vi "PXI_Host_U16_Read_NewMethod_Benchmark.vi"() -> ()   [LabVIEW 2018]
uses:
  <vilib>/Platform/TimedLoop/XDataNode/timing_clust.ctl
  <vilib>/Platform/TimedLoop/XDataNode/nitl_modes.ctl
  <vilib>/Platform/TimedLoop/XDataNode/wakeup.ctl
  cRIO RT/FPGA Bitfile Register Operations/Scalar IO Operations/Read Methods/Read Data Register/Instances/Read U16.vi
  cRIO RT/FPGA Bitfile Register Operations/Scalar IO Operations/Utilities/Find Register Offset.vi
  cRIO RT/FPGA Bitfile Register Operations/Scalar IO Operations/SubVIs/Check Register Data Store.vi
  cRIO RT/FPGA Bitfile Register Operations/Scalar IO Operations/Error Handling/Error 6001.vi
  cRIO RT/FPGA Bitfile Register Operations/Scalar IO Operations/Error Handling/Error 6000.vi
  cRIO RT/FPGA Bitfile Register Operations/Scalar IO Operations/Error Handling/Error 6002.vi
  cRIO RT/FPGA Bitfile Register Operations/Scalar IO Operations/Error Handling/Error 6003.vi
  <vilib>/FPGAPlugInAG/Dynamic/niLvFpga_Close_Dynamic.vi
  <vilib>/platform/TimedLoop/XDataNode/XDataNode.xnode
  <vilib>/rvi/interface/nirviCloseFPGA/nirviCloseFPGA.xnode
  cRIO RT/FPGA Bitfile Register Operations/Scalar IO Operations/FPGA Register IO.lvlib
  <vilib>/Platform/TimedLoop/XDataNode/XDNodeRunTimeDep.lvlib
panel:
  out "Standard Dev":dbl
  out "Execution time (s)":dbl
  out "Maximum(s)":dbl
  out "Waveform Graph":dbl[](graph)
  out "Value out":i8
  out "error out":errorcluster
  # "Recorded time"
  # "3.37551E-5"
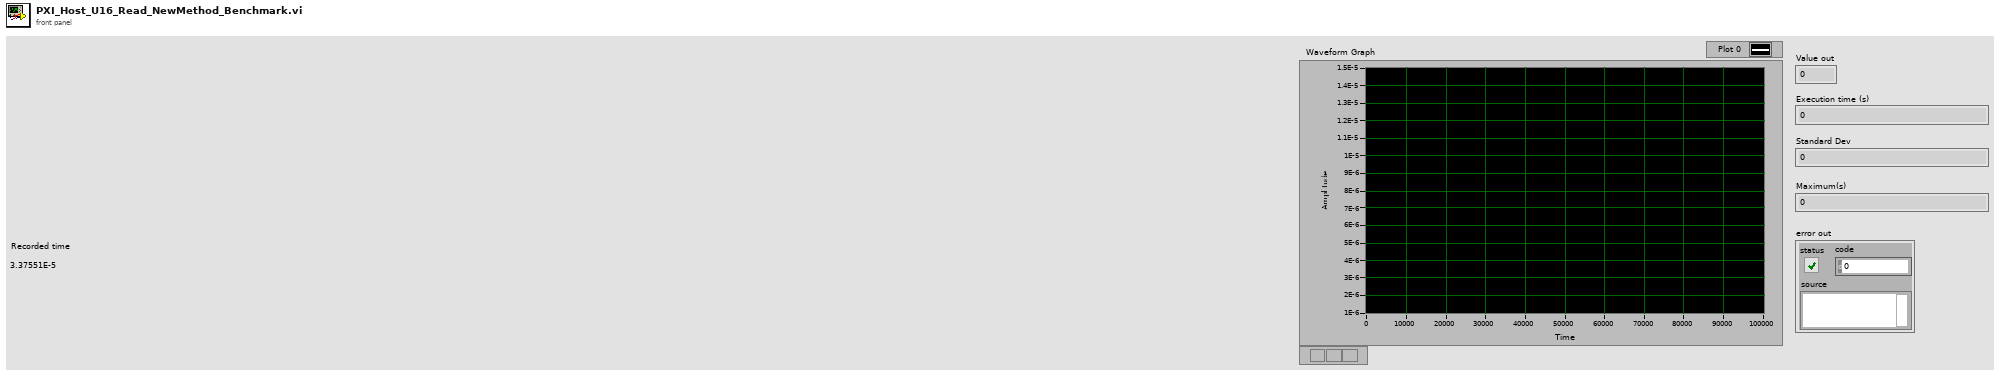
[diagram p1: front panel]
types:
  T1 = typedef "XDNodeRunTimeDep.lvlib/timing_clust.ctl" = cluster{"Expected End [f-1]":u64, "Actual End [f-1]":u64, "Finished Late? [f-1]":bool, "Expected End [i-1]":u64, "Actual End [i-1]":u64, "Finished Late? [i-1]":bool, "Expected Start [i]":u64, "Actual Start [i]":u64, "Expected Start [f]":u64, "Actual Start [f]":u64, "Source Name":string, "Structure Name":string, "Period":i64, "Deadline":i64, "Offset":i64, "Start":i64, "Priority":i32, "Timeout":i32, "Mode":T2, "Wakeup Reason":T3, "Error":errorcluster, "Source Type":string, "Secondary Source Type":string, "Global End Time":u64, "Global Start Time":u64, "Frame Duration":u64, "Iteration Duration":u64, "Assigned CPU":i32, "I/O Scan Engine Mode":u32}
  T2 = typedef "XDNodeRunTimeDep.lvlib/nitl_modes.ctl" = enum32{"No Change", "Process missed periods, maintain original phase", "Discard missed periods, maintain original phase", "Process missed periods, ignore original phase", "Discard missed periods, ignore original phase"}
  T3 = typedef "XDNodeRunTimeDep.lvlib/wakeup.ctl" = enum32{"Normal", "Aborted", "Asynchronous wakeup", "Timing source error", "Timed loop error", "Timeout"}
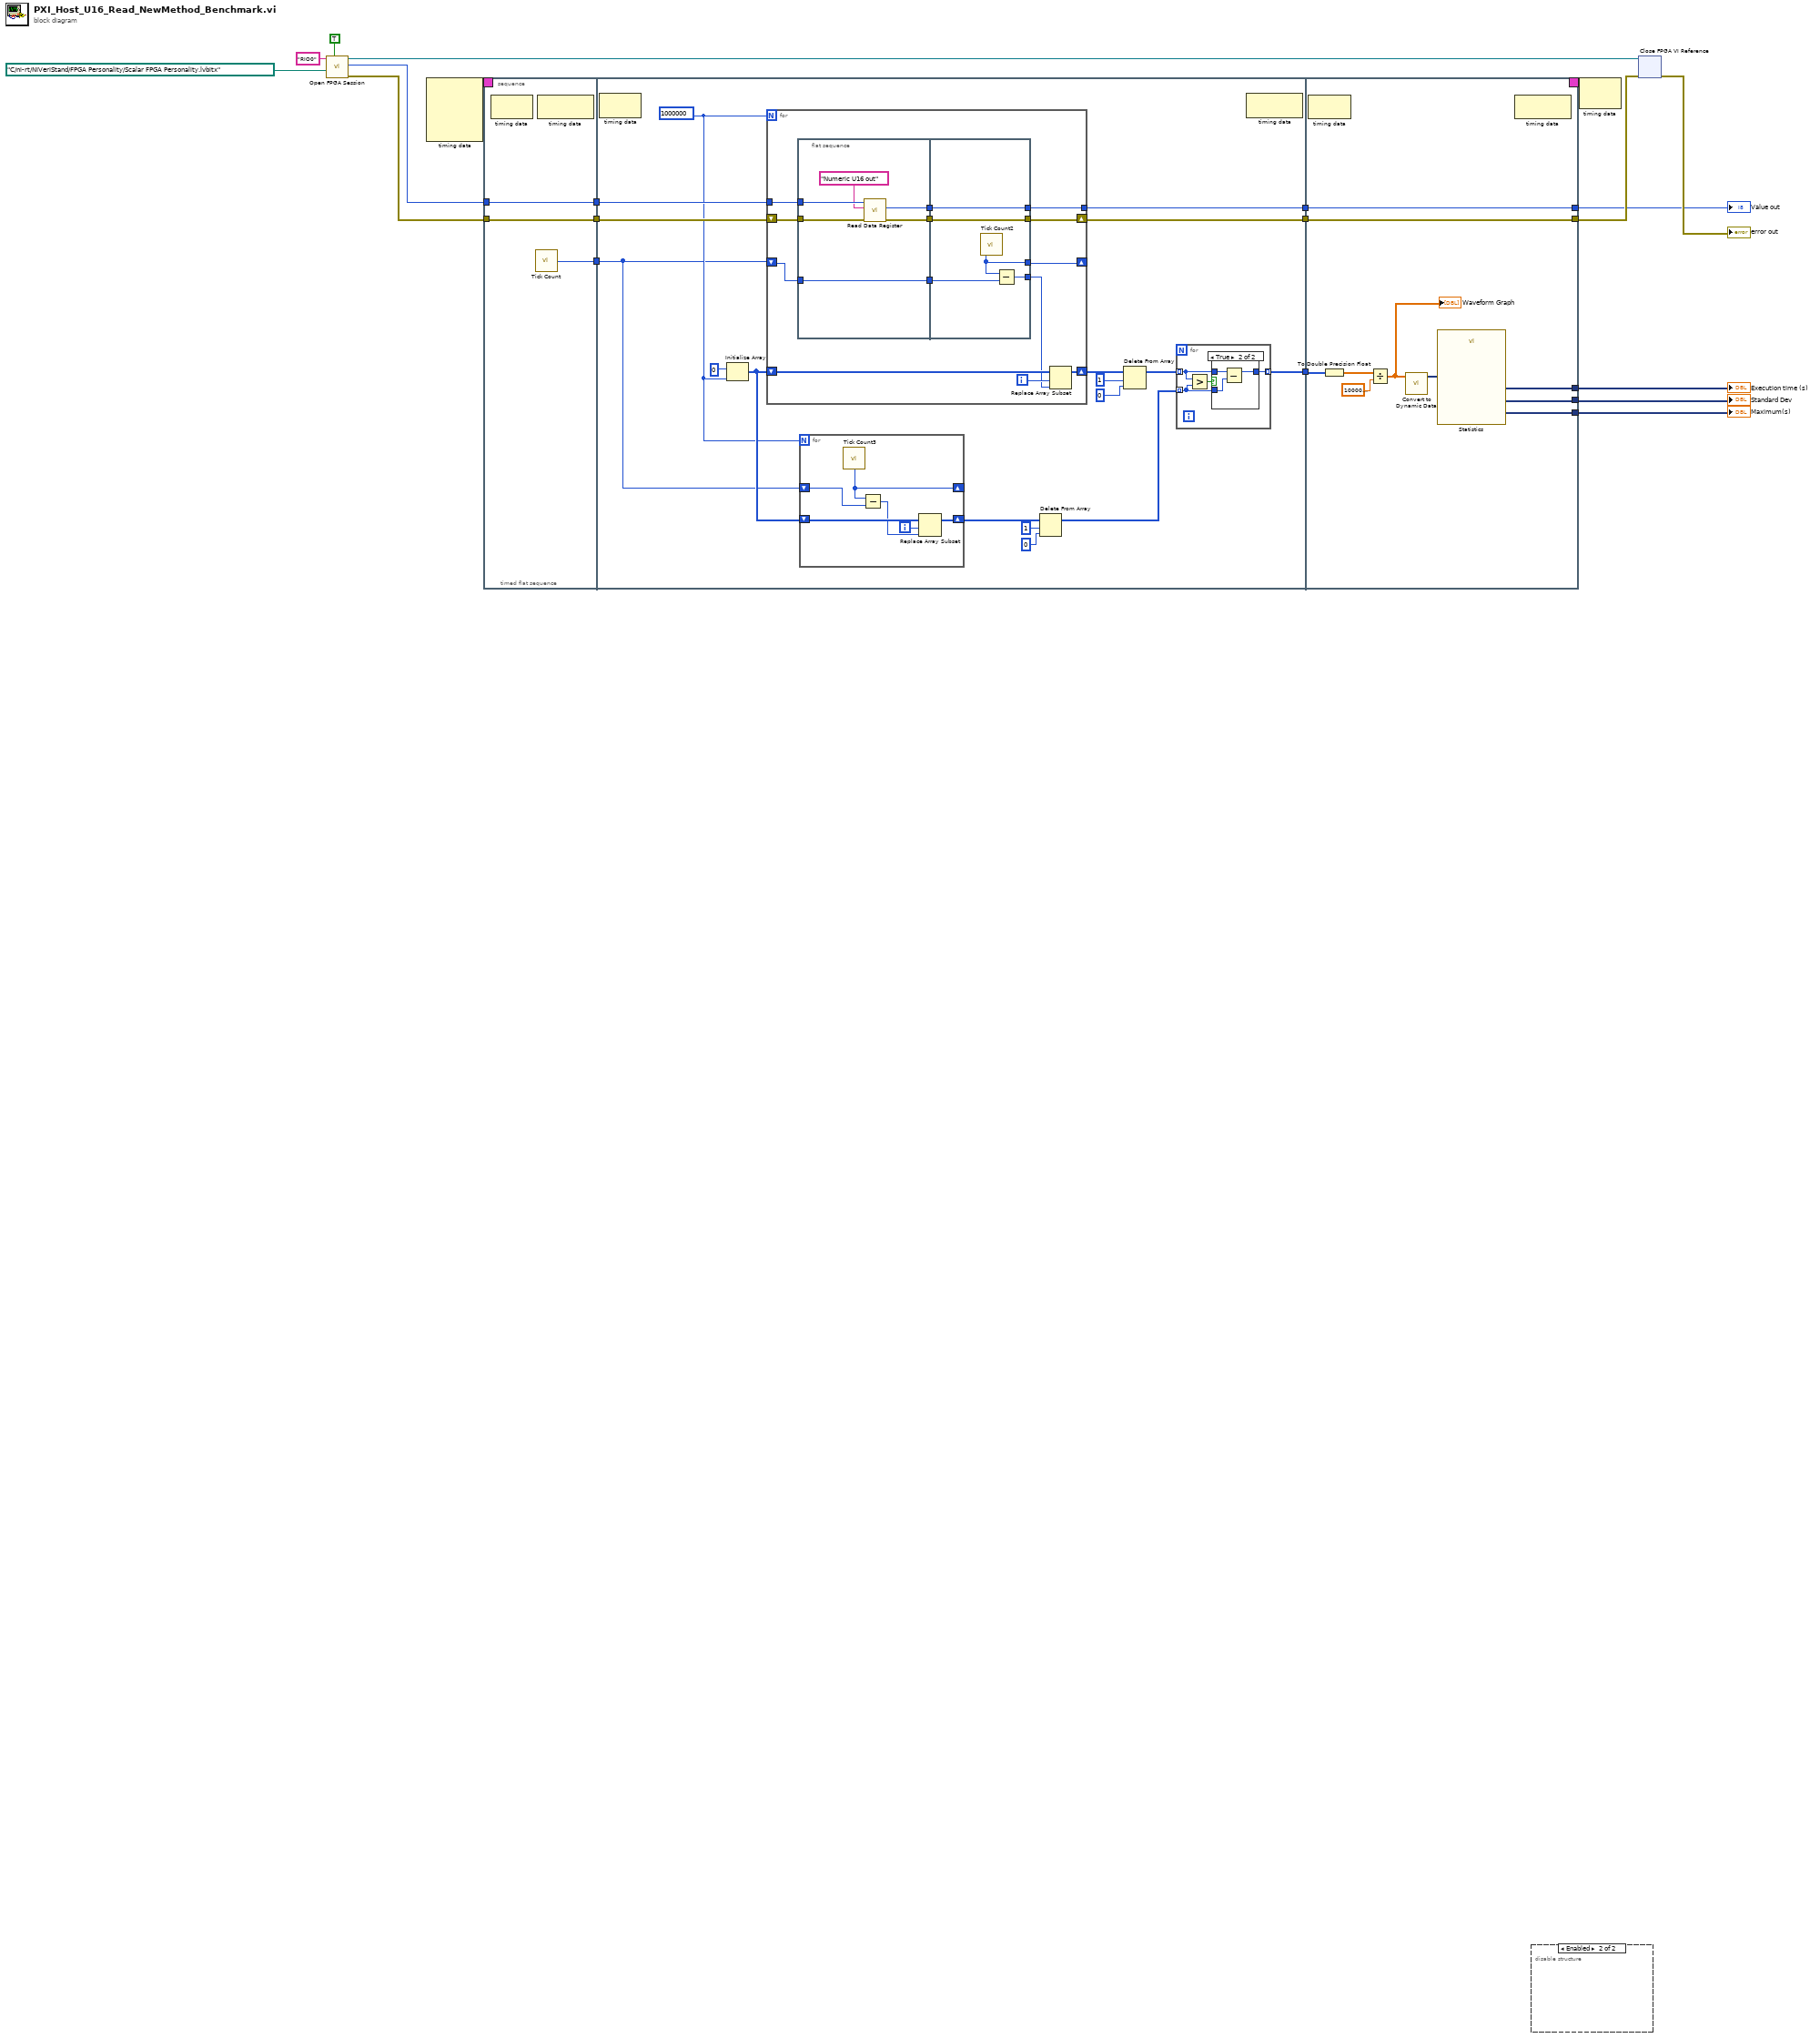
[diagram p0: block diagram]
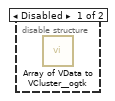
[diagram p3: hidden frame]
diagram:
  n1 = call "Open FPGA Session.vi"("run when loaded (T)"=TRUE, "bitfile path"=path "C:/ni-rt/NIVeriStand/FPGA Personality/Scalar FPGA Personality.lvbitx", "device address"="RIO0") -> ("error out"=w10:errorcluster, "session out"=w14:u32, "bitfile reference out"=w9:refnum<k20>)  [unwired: 6 in]
  n2 = node-c288() -> (w5:T1)  [unwired: 4 in]
  n3 = timed-sequence {
    timing: w5 -> [_]
    timing-out: [_] -> w4
    tunnel: w14 -> [w27]
    tunnel: w10 -> [w26]
    tunnel: [w25] -> w8
    tunnel: [w24] -> w6
    tunnel: [w17] -> w3
    tunnel: [w16] -> w2
    tunnel: [w15] -> w1
    n4 = timed-flat-sequence {
      tunnel: w26 -> [w29]
      tunnel: w27 -> [w30]
      tunnel: [w30] -> w23
      tunnel: [w29] -> w22
      tunnel: [w28] -> w21
      tunnel: w23 -> [w49]
      tunnel: w22 -> [w48]
      tunnel: w21 -> [w33]
      tunnel: [w47] -> w20
      tunnel: [w46] -> w19
      tunnel: [w34] -> w18
      tunnel: [w98] -> w24
      tunnel: [w99] -> w25
      tunnel: w20 -> [w99]
      tunnel: w19 -> [w98]
      tunnel: w18 -> [w93]
      tunnel: [w92] -> w17
      tunnel: [w91] -> w16
      tunnel: [w90] -> w15
      frame #0 {
        n5 = node-c288() -> ()  [unwired: 1 in, 1 out]
        n6 = call "Tick Count"() -> ("Tick Count(Ticks)"=w28:u32)
        n7 = node-c288() -> ()  [unwired: 1 in, 1 out]
      }
      frame #1 {
        w37 = 1000000
        n8 = node-c288() -> ()  [unwired: 1 in, 1 out]
        n9 = Initialize Array(u32 0 ("Tick Count(uSec)"), w37) -> (w38:u32[])
        n10 = for {
          N: w37 -> [_]
          tunnel: w49 -> [w74]
          tunnel: [w71] -> w46
          shift-right: [w72] -> w47
          shift-left: w48 -> [w73]
          shift-right: [w66] -> _
          shift-left: w33 -> [w69]
          shift-right: [w65] -> w43
          shift-left: w38 -> [w68]
          i -> [w67]
          n11 = flat-sequence {
            tunnel: [w80] -> w76
            tunnel: [w79] -> w75
            tunnel: w74 -> [w82]
            tunnel: w73 -> [w81]
            tunnel: [w77] -> w70
            tunnel: w69 -> [w77]
            tunnel: [w87] -> w64
            tunnel: w76 -> [w86]
            tunnel: [w86] -> w72
            tunnel: w75 -> [w85]
            tunnel: [w85] -> w71
            tunnel: w70 -> [w84]
            tunnel: [w83] -> w66
            frame #0 {
              n12 = call-poly "Read Data Register.vi"("error in"=w81, "register name"="Numeric U16 out", "session in"=w82) -> ("error out"=w80:errorcluster, "value out"=w79:u16)  [unwired: 6 in, 1 out]
            }
            frame #1 {
              n13 = call "Tick Count2"() -> ("Tick Count(Ticks)"=w83:u32)
              n14 = Subtract(x=w83, y=w84) -> (x-y=w87:u32)
            }
          }
          n15 = Replace Array Subset(array=w68, new element=w64, index=w67) -> (w65:u32[])
        }
        n16 = for {
          N: w37 -> [_]
          shift-right: [w58] -> w39
          shift-left: w38 -> [w61]
          shift-right: [w63] -> _
          shift-left: w33 -> [w62]
          i -> [w59]
          n17 = call "Tick Count3"() -> ("Tick Count(Ticks)"=w63:u32)
          n18 = Subtract(x=w63, y=w62) -> (x-y=w60:u32)
          n19 = Replace Array Subset(array=w61, new element=w60, index=w59) -> (w58:u32[])
        }
        n20 = Delete From Array(array=w39, length=1, index=0) -> (array with subset deleted=w35:u32[])  [unwired: 1 out]
        n21 = Delete From Array(array=w43, length=1, index=0) -> (array with subset deleted=w36:u32[])  [unwired: 1 out]
        n22 = for {
          tunnel: [w53] -> w34 mode=indexing
          tunnel: w36 -> [w52] mode=indexing
          tunnel: w35 -> [w51] mode=indexing
          n23 = Greater?(x=w52, y=w51) -> (0:w50:bool)
          n24 = case shown="True" w50 {
            tunnel: w52 -> [w54 w57]
            tunnel: w51 -> [_ w56]
            tunnel: [w54 w55] -> w53
            frame False {
            }
            frame True {
              n25 = Subtract(x=w57, y=w56) -> (x-y=w55:u32)
            }
          }
        }
        n26 = node-c288() -> ()  [unwired: 1 in, 1 out]
      }
      frame #2 {
        n27 = node-c288() -> ()  [unwired: 1 in, 1 out]
        n28 = To Double Precision Float(number=w93) -> (double precision float=w97:dbl[])
        n29 = Divide(x=w97, y=1000000000.0) -> (x/y=w94:dbl[])
        "Waveform Graph" <- w94
        n30 = call "Convert to Dynamic Data"("Array"=w94) -> ("Dynamic Data Type"=w95:dynamicdata)  [unwired: 3 in]
        n31 = call "Statistics"("Signals"=w95) -> ("Standard Dev"=w91:dynamicdata, "Arithmetic Mean"=w92:dynamicdata, "Maximum"=w90:dynamicdata)  [unwired: 23 in, 1 out]
        n32 = node-c288() -> ()  [unwired: 1 in, 1 out]
      }
    }
  }
  "Value out" <- w6
  "Maximum(s)" <- w1
  "Execution time (s)" <- w3
  "Standard Dev" <- w2
  n33 = disable-structure shown="Enabled" {
    frame Disabled {
      n34 = call <userlib>:"Array of VData to VCluster__ogtk.vi"() -> ()  [unwired: 10 in, 2 out]
    }
    frame Enabled {
    }
  }
  n35 = node-c288(w4) -> ()  [unwired: 1 out]
  n36 = xnode "Close FPGA VI Reference"("FPGA VI Reference In"=w9, "error in"=w8) -> ("error out"=→"error out":errorcluster)
